vi "ROI_mean_calculator.vi"() -> ()   [LabVIEW 2018]
uses:
  <vilib>/vision/NI_Vision_Development_Module.lvlib
panel:
  out "filenames":string[](array[string])
  out "Image 2":T1(plugin-control)
  in  "Slide":dbl(slide) scale=0.0..800.0
  in  "Stop":bool
  out "Numeric":i32
  out "Mean":sgl[](array[numeric])
  out "Mean Intensity ROI":sgl[](graph)
  out "Progress":u8(slide) scale=0.0..100.0
  out "Image":T1(plugin-control)
  in  "stop":bool
  in  "Image path (dialog if empty)":path
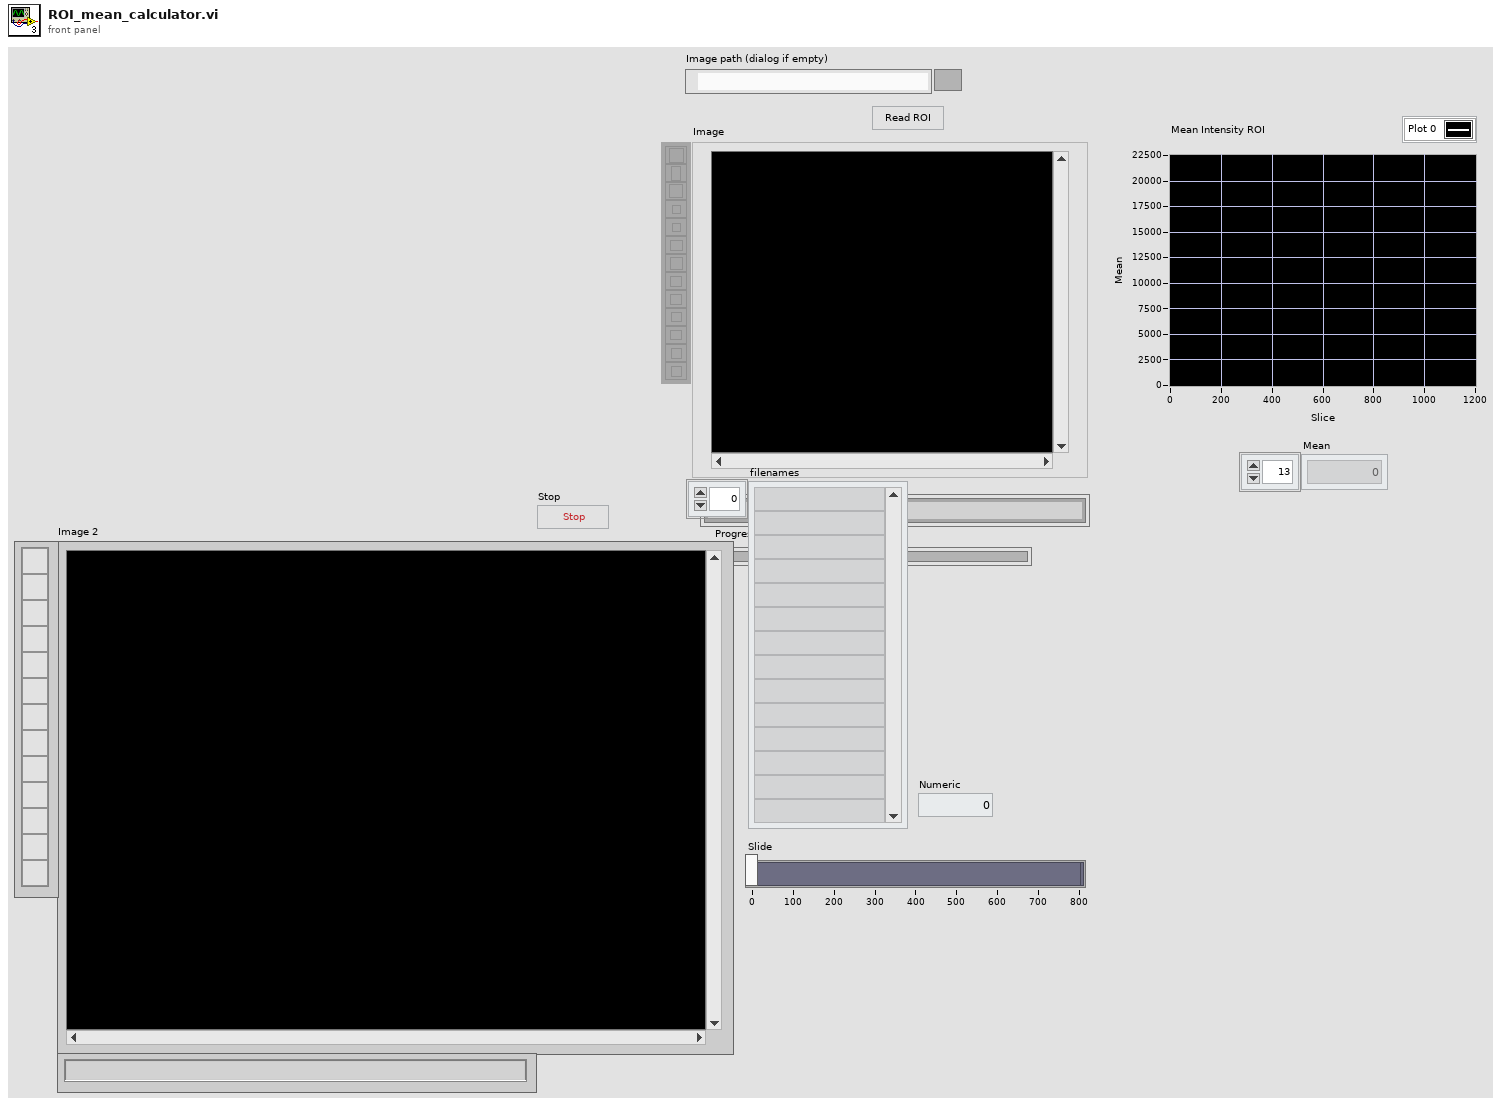
[diagram p1: front panel]
types:
  T1 = typedef "IMAQ Image.ctl" = refnum<image>
  T2 = typedef "Image Type" = u32
  T3 = cluster{"Global Rectangle":i32[], "Contours":cluster{"Contour Type":u32, "ROI Type":u32, "Points":i32[]}[]}
  T4 = cluster{"Mean Intensity":sgl, "Standard  Deviation":sgl, "Minimum Intensity":sgl, "Maximum Intensity":sgl}
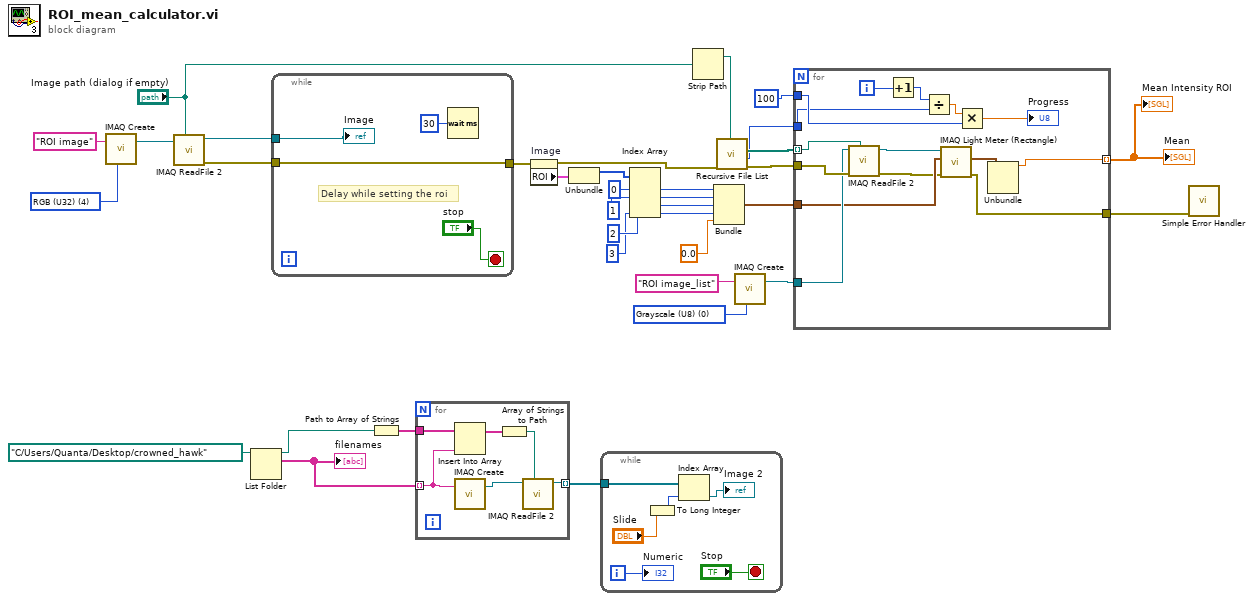
[diagram p0: block diagram]
diagram:
  w13 = T2 0 items=["Grayscale (U8)", "Grayscale (I16)", "Grayscale (SGL)", "Complex (CSG)", "RGB (U32)", "HSL (U32)", "RGB (U64)", "Grayscale (U16)"] ("Image Type")
  w33 = T2 4 items=["Grayscale (U8)", "Grayscale (I16)", "Grayscale (SGL)", "Complex (CSG)", "RGB (U32)", "HSL (U32)", "RGB (U64)", "Grayscale (U16)"] ("Image Type")
  n1 = call "IMAQ Create"("Image Name"="ROI image", "Image Type"=w33) -> ("New Image"=w35:T1)  [unwired: 3 in, 1 out]
  n2 = call "IMAQ ReadFile 2"("File Path"="Image path (dialog if empty)", "Image"=w35) -> ("error out"=w31:errorcluster, "Image Out"=w32:T1)  [unwired: 5 in, 3 out]
  n3 = List Folder(path=path "C:/Users/Quanta/Desktop/crowned_hawk") -> (path out=w4:path, filenames=w2:string[])  [unwired: 3 in, 2 out]
  "filenames" <- w2
  n4 = while {
    tunnel: w32 -> [w36]
    tunnel: [w37] -> w30
    tunnel: w31 -> [w37]
    stop <- "stop" stop-if-true
    # "Delay while setting the roi"
    n5 = Wait (ms)(milliseconds to wait=u32 30) -> ()  [unwired: 1 out]
    "Image" <- w36
  }
  n6 = Path to Array of Strings(0:w4) -> (2:w3:string[])  [unwired: 1 out]
  n7 = for {
    tunnel: w2 -> [w42] mode=indexing
    tunnel: [w44] -> w1 mode=indexing
    tunnel: w3 -> [w43]
    n8 = Insert Into Array(array=w43, new element=w42) -> (w41:string[])  [unwired: 1 in]
    n9 = call "IMAQ Create"("Image Name"=w42) -> ("New Image"=w45:T1)  [unwired: 4 in, 1 out]
    n10 = Array of Strings to Path(0:w41) -> (2:w40:path)  [unwired: 1 in]
    n11 = call "IMAQ ReadFile 2"("File Path"=w40, "Image"=w45) -> ("Image Out"=w44:T1)  [unwired: 5 in, 4 out]
  }
  n12 = property on="Image" class="ImageControl"(error in=w30) -> (error out=w16:errorcluster, "ROI"=w25:T3)  [unwired: 1 in, 1 out]
  n13 = Unbundle(w25) -> ("Global Rectangle"=w24:i32[])  [unwired: 1 out]
  n14 = while {
    tunnel: w1 -> [w51]
    i -> [w46]
    stop <- "Stop" stop-if-true
    n15 = To Long Integer(number="Slide") -> (32bit integer=w48:i32)
    n16 = Index Array(array=w51, index=w48) -> (element=→"Image 2":T1)
    "Numeric" <- w46
  }
  n17 = Index Array(array=w24, index #1=0 ("index"), index #2=1 ("index"), index #3=2 ("index"), index #4=3 ("index")) -> (element #1=w23:i32, element #2=w22:i32, element #3=w21:i32, element #4=w20:i32)
  n18 = Strip Path(path="Image path (dialog if empty)") -> (stripped path=w17:path)  [unwired: 1 out]
  n19 = Bundle(w23, w22, w21, w20, 0.0) -> (w8:cluster{i32, i32, i32, i32, dbl})  [unwired: 1 in]
  n20 = call <vilib>:"Recursive File List.vi"("error in (no error)"=w16, "Folder Path"=w17) -> ("error out"=w15:errorcluster, "Number of Files"=w9:i32, "All Files in Dir"=w11:path[])  [unwired: 5 in, 2 out]
  n21 = call "IMAQ Create"("Image Name"="ROI image_list", "Image Type"=w13) -> ("New Image"=w12:T1)  [unwired: 3 in, 1 out]
  n22 = for {
    tunnel: w15 -> [w66]
    tunnel: w12 -> [w65]
    tunnel: w11 -> [w64] mode=indexing
    tunnel: 100 -> [w60]
    tunnel: w9 -> [w59]
    tunnel: w8 -> [w58]
    tunnel: [w52] -> w7 mode=indexing
    tunnel: [w53] -> w6
    i -> [w63]
    n23 = call "IMAQ ReadFile 2"("File Path"=w64, "error in (no error)"=w66, "Image"=w65) -> ("error out"=w54:errorcluster, "Image Out"=w57:T1)  [unwired: 4 in, 3 out]
    n24 = Increment(x=w63) -> (x+1=w62:i32)
    n25 = Divide(x=w62, y=w59) -> (x/y=w61:dbl)
    n26 = call "IMAQ Light Meter (Rectangle)"("error in (no error)"=w54, "Rectangle"=w58, "Image"=w57) -> ("error out"=w53:errorcluster, "Gray Level Intensities"=w56:T4)  [unwired: 4 in, 3 out]
    n27 = Multiply(x=w61, y=w60) -> (x*y=→"Progress":dbl)
    n28 = Unbundle(w56) -> ("Mean Intensity"=w52:sgl)  [unwired: 3 out]
  }
  "Mean Intensity ROI" <- w7
  "Mean" <- w7
  n29 = call <vilib>:"Simple Error Handler.vi"("error in (no error)"=w6) -> ()  [unwired: 4 in, 5 out]
